vi "dfd_NIDFDTYP_H.vi"() -> ()   [LabVIEW 2017, in "NI_DigFilterTemp.lvlib"]
uses:
  <vilib>/addons/Digital Filter Design/NI_DigFilterTemp.lvlib
panel:
  in  "String":string="/* ======================================================================\n * Title:     nidfdtyp.h                                                 \n *                                                                       \n * Purpose:                                                              \n *            Define the basic datatypes used in the C source files,     \n * which are generated by Digital Filter Design toolkit.                 \n *                                                                       \n * Copyright 2008 National Instruments Corporation. All rights reserved. \n * ======================================================================\n */\n\n#ifndef __NI_DFD_TYPE_H__\n#define __NI_DFD_TYPE_H__\n\ntypedef short I16;\ntypedef long I32;\ntypedef unsigned long U32;\n\n#endif //#ifndef __NI_DFD_TYPE_H__\n"
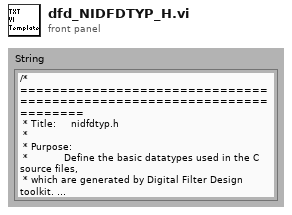
[diagram p1: front panel]
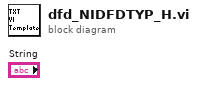
[diagram p0: block diagram]
diagram:
